vi "Determine Clicked Array Element Index - Determine Array and Scrollbar Properties.vi"(8 "error in (no error)":errorcluster, 10 "Coords of Click":T1, 11 "Array Reference":refnum<vi>) -> (0 "error out":errorcluster, 1 "Scrollbar Properties":T2, 2 "Array Properties":T5, 3 "dup Array Reference":refnum<vi>, 5 "Array Label":string)   [LabVIEW 2021, in "Arrays.lvlib"]
doc: "Determine Clicked Array Element Index - Determine Array and Scrollbar Properties.vi\n\nDescription:\nThis VI determines multiple properties of the array and scrollbars of the array specified by the Array Reference input.\n\nIf no caption has been created for the array of interest, instruct the user how to correct the issue.\n\nInputs:\nArray Reference - Reference to the array to operate on.\n\nCoords of Click - The screen coordinates of the click within the array. These values are used to determine if the click occurred on the selected item.\n\nerror in - Standard error cluster.\n\nOutputs:\ndup Array Reference - Dup reference to the array to operate on.\n\nArray Properties - Cluster containing the array properties of the array specified by the Array Reference input.\n\nScrollbar Properties - Cluster containing the scrollbar properties of the array specified by the Array Reference input.\n\nerror out - standard error cluster.\n\nDeveloped By:\nMark.ridgley\nMark.Ridgley_LabVIEW.Developer@comcast.net"
uses:
  Arrays.lvlib
  <vilib>/Utility/miscctls.llb/LVBoundsTypeDef.ctl
  <vilib>/Utility/miscctls.llb/LVPositionTypeDef.ctl
  <vilib>/Utility/miscctls.llb/LVPoint32TypeDef.ctl
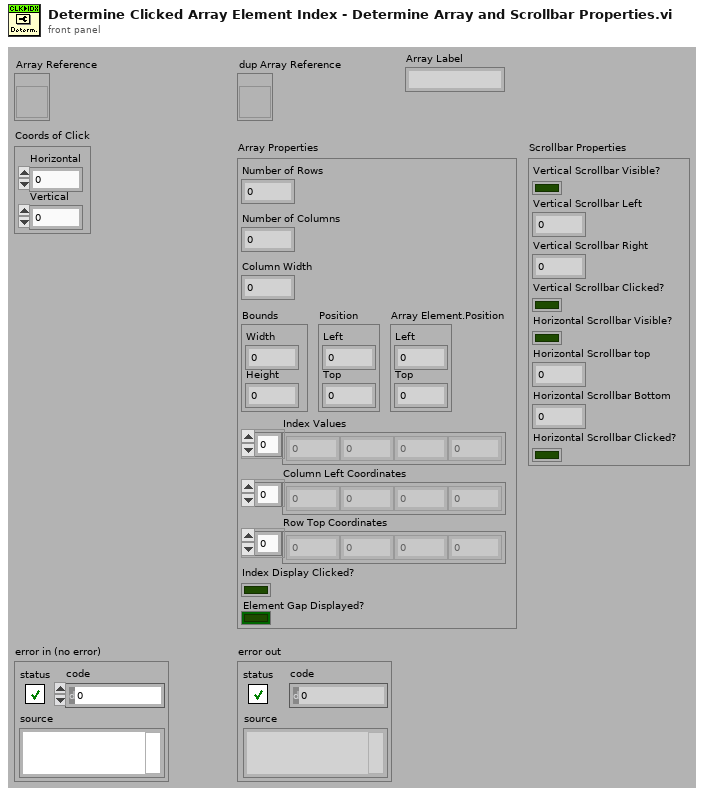
[diagram p1: front panel]
types:
  T1 = typedef "LVPoint32TypeDef.ctl" = cluster{"Horizontal":i32, "Vertical":i32}
  T2 = cluster{"Vertical Scrollbar Visible?":bool, "Vertical Scrollbar Left":i32, "Vertical Scrollbar Right":i32, "Vertical Scrollbar Clicked?":bool, "Horizontal Scrollbar Visible? ":bool, "Horizontal Scrollbar top":i32, "Horizontal Scrollbar Bottom":i32, "Horizontal Scrollbar Clicked?":bool}
  T3 = typedef "LVBoundsTypeDef.ctl" = cluster{"Width":u32, "Height":u32}
  T4 = typedef "LVPositionTypeDef.ctl" = cluster{"Left":i32, "Top":i32}
  T5 = cluster{"Number of Rows":u32, "Number of Columns":u32, "Column Width":u32, "Bounds":T3, "Position":T4, "Array Element.Position":T4, "Index Values":u32[], "Column Left Coordinates":i32[], "Row Top Coordinates":i32[], "Index Display Clicked?":bool, "Element Gap Displayed?":bool}
  T6 = enum16{"Horizontal Scrollbar", "Vertical Scrollbar"}
  T7 = enum16{"Horizontal Scrollbar", "Vertical Scrollbar", "Index Display"}
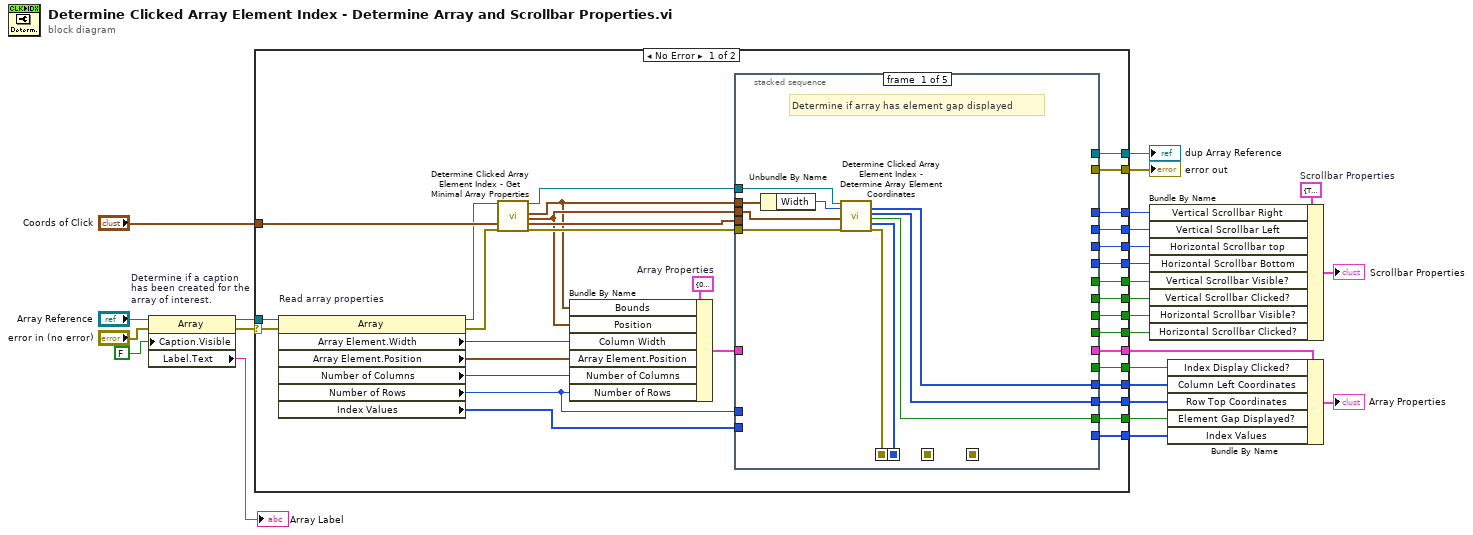
[diagram p0: block diagram]
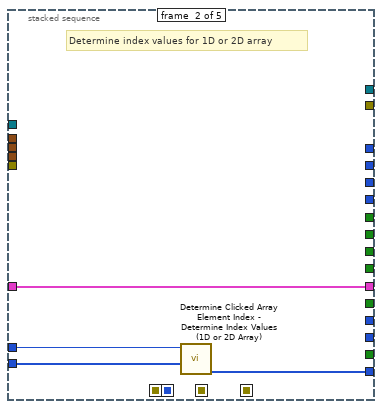
[diagram p2: hidden frame]
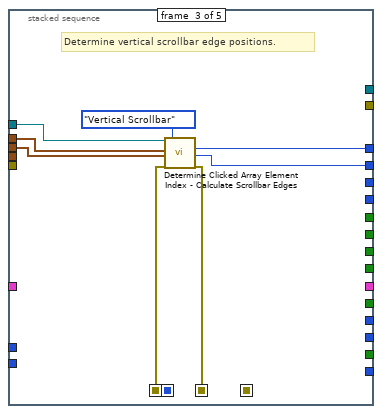
[diagram p3: hidden frame]
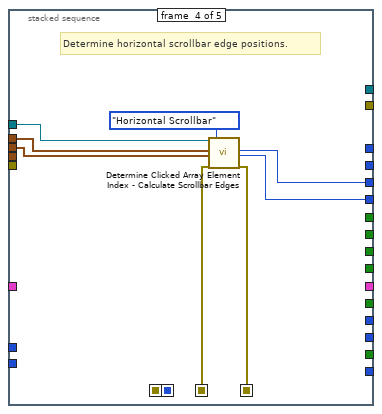
[diagram p4: hidden frame]
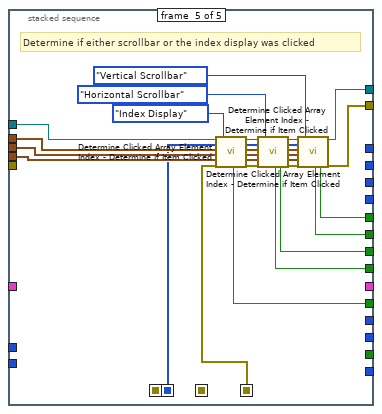
[diagram p5: hidden frame]
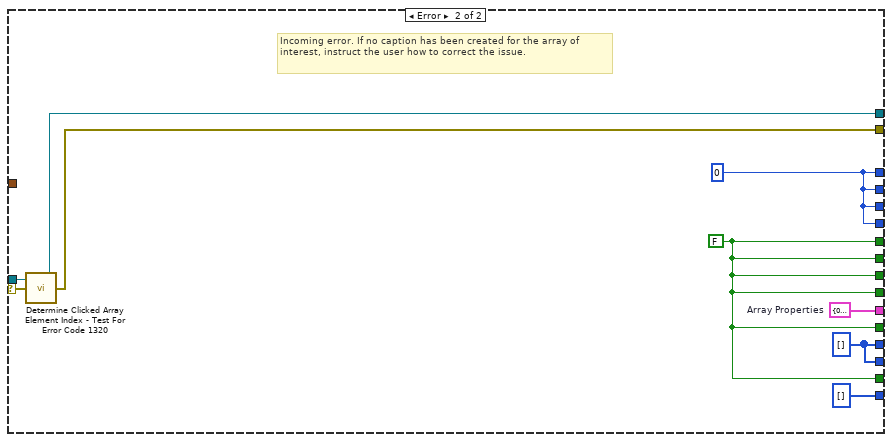
[diagram p6: hidden frame]
diagram:
  w2 = T2 {"Vertical Scrollbar Visible?"=TRUE, "Vertical Scrollbar Left"=0, "Vertical Scrollbar Right"=0, "Vertical Scrollbar Clicked?"=FALSE, "Horizontal Scrollbar Visible? "=TRUE, "Horizontal Scrollbar top"=0, "Horizontal Scrollbar Bottom"=0, "Horizontal Scrollbar Clicked?"=TRUE}  # Scrollbar Properties
  n1 = property on="Determine if a caption has been created for the array of interest." class="Array"(reference="Array Reference", error in="error in (no error)", "Caption.Visible"=FALSE) -> (reference out=w7:refnum<vi>, error out=w8:errorcluster, "Label.Text"=→"Array Label":string)
  n2 = case shown="No Error" w8 {
    selector: w8 -> [w31 w122]
    tunnel: "Coords of Click" -> [w59 _]
    tunnel: [w58 u32[] [] ("Column Left Coordinates")] -> w24
    tunnel: w7 -> [w57 w125]
    tunnel: [w54 w124] -> w23
    tunnel: [w53 w124] -> w22
    tunnel: [w52 w124] -> w21
    tunnel: [w51 w124] -> w20
    tunnel: [w50 w124] -> w19
    tunnel: [w47 w125] -> w18
    tunnel: [w46 w118] -> w17
    tunnel: [w45 w118] -> w16
    tunnel: [w43 w123] -> w15
    tunnel: [w42 w123] -> w14
    tunnel: [w41 w124] -> w13
    tunnel: [w33 w119] -> w12
    tunnel: [w32 w121] -> w11
    tunnel: [w28 w118] -> w4
    tunnel: [w27 w118] -> w3
    frame No Error {
      w29 = T5 {"Number of Rows"=0, "Number of Columns"=0, "Column Width"=0, "Bounds"={"Width"=0, "Height"=0}, "Position"={"Left"=0, "Top"=0}, "Array Element.Position"={"Left"=0, "Top"=0}, "Index Values"=[], "Column Left Coordinates"=[], "Row Top Coordinates"=[], "Index Display Clicked?"=FALSE, "Element Gap Displayed?"=FALSE}  # Array Properties
      n3 = property on="Read array properties" class="Array"(reference=w57, error in=w31) -> (reference out=w55:refnum<vi>, error out=w56:errorcluster, "Array Element.Width"=w30:u32, "Array Element.Position"=w37:T4, "Number of Columns"=w35:u32, "Number of Rows"=w36:u32, "Index Values"=w38:u32[])
      n4 = call "Determine Clicked Array Element Index - Get Minimal Array Properties.vi"("Array Reference"=w55, "Coords of Click"=w59, "error in (no error)"=w56) -> ("dup Array Reference"=w44:refnum<vi>, "Minimal Array Properties.Bounds"=w39:T3, "Minimal Array Properties.Position"=w40:T4, "dup Coords of Click"=w49:T1, "error out"=w48:errorcluster)  [unwired: 12 in]
      n5 = Bundle By Name(cluster=w29, "Bounds"=w39, "Position"=w40, "Column Width"=w30, "Array Element.Position"=w37, "Number of Columns"=w35, "Number of Rows"=w36) -> (w34:T5)
      n6 = stacked-sequence {
        seq-local: [w65 _ _ _ _] -> [_ _ _ _ w93]
        seq-local: [w62 _ _ _ _] -> [_ _ w78 _ _]
        seq-local: [_ _ w77 _ _] -> [_ _ _ w88 _]
        seq-local: [_ _ _ w87 _] -> [_ _ _ _ w90]
        tunnel: [_ w70 _ _ _] -> w58
        tunnel: w38 -> [_ w73 _ _ _]
        tunnel: [_ _ _ _ w114] -> w54
        tunnel: [_ _ _ _ w113] -> w53
        tunnel: [_ _ _ _ w112] -> w52
        tunnel: [_ _ _ _ w111] -> w51
        tunnel: [_ _ _ _ w110] -> w50
        tunnel: w49 -> [_ _ _ _ w97]
        tunnel: w48 -> [w63 _ _ _ _]
        tunnel: [_ _ _ _ w91] -> w47
        tunnel: [_ _ _ _ w92] -> w32
        tunnel: [_ _ w80 _ _] -> w46
        tunnel: [_ _ w79 _ _] -> w45
        tunnel: w39 -> [w61 _ w76 w84 w96]
        tunnel: w36 -> [_ w72 _ _ _]
        tunnel: w40 -> [w64 _ w75 w83 w95]
        tunnel: w44 -> [w69 _ w81 w89 w94]
        tunnel: [w68 _ _ _ _] -> w43
        tunnel: [w67 _ _ _ _] -> w42
        tunnel: [w66 _ _ _ _] -> w41
        tunnel: w34 -> [_ w71 _ _ _]
        tunnel: [_ w71 _ _ _] -> w33
        tunnel: [_ _ _ w86 _] -> w28
        tunnel: [_ _ _ w85 _] -> w27
        frame #0 {
          # "Determine if array has element gap displayed"
          n7 = Unbundle By Name(w61) -> ("Width"=w60:u32)
          n8 = call "Determine Clicked Array Element Index - Determine Array Element Coordinates.vi"("Array Reference"=w69, "Minimal Array Properties.Bounds.Width"=w60, "Minimal Array Properties.Position"=w64, "error in (no error)"=w63) -> ("Column Left Coordinates"=w68:i32[], "Row Top Coordinates"=w67:i32[], "Array has element gap?"=w66:bool, "Un-gapped left coordinates"=w65:i32[], "error out"=w62:errorcluster)  [unwired: 10 in, 1 out]
        }
        frame #1 {
          # "Determine index values for 1D or 2D array"
          n9 = call "Determine Clicked Array Element Index - Determine Index Values (1D or 2D Array).vi"("Array Property.Index Values"=w73, "Array Property.Number of Rows"=w72) -> ("Index Values (1D or 2D Array)"=w70:u32[])  [unwired: 9 in]
        }
        frame #2 {
          # "Determine vertical scrollbar edge positions."
          n10 = call "Determine Clicked Array Element Index - Calculate Scrollbar Edges.vi"("Array Reference"=w81, "Minimal Array Properties.Bounds"=w76, "Minimal Array Properties.Position"=w75, "error in (no error)"=w78, "Select Item"=T6."Vertical Scrollbar") -> ("Minimum Scrollbar Edge"=w79:i32, "Maximum Scrollbar Edge"=w80:i32, "error out"=w77:errorcluster)  [unwired: 11 in, 1 out]
        }
        frame #3 {
          # "Determine horizontal scrollbar edge positions."
          n11 = call "Determine Clicked Array Element Index - Calculate Scrollbar Edges.vi"("Array Reference"=w89, "Minimal Array Properties.Bounds"=w84, "Minimal Array Properties.Position"=w83, "error in (no error)"=w88, "Select Item"=T6."Horizontal Scrollbar") -> ("Minimum Scrollbar Edge"=w86:i32, "Maximum Scrollbar Edge"=w85:i32, "error out"=w87:errorcluster)  [unwired: 11 in, 1 out]
        }
        frame #4 {
          # "Determine if either scrollbar or the index display was clicked"
          n12 = call "Determine Clicked Array Element Index - Determine if Item Clicked.vi"("Array Reference"=w94, "Un-gapped left coordinates"=w93, "Minimal Array Properties.Bounds"=w96, "Minimal Array Properties.Position"=w95, "Coords of Click"=w97, "error in (no error)"=w90, "Select Item"=T7."Index Display") -> ("Item Clicked?"=w114:bool, "dup Array Reference"=w117:refnum<vi>, "dup Un-gapped left coordinates"=w102:i32[], "dup Minimal Array Properties.Bounds"=w108:T3, "dup Minimal Array Properties.Position"=w104:T4, "dup Coords of Click"=w103:T1, "error out"=w109:errorcluster)  [unwired: 5 in, 1 out]
          n13 = call "Determine Clicked Array Element Index - Determine if Item Clicked.vi"("Array Reference"=w117, "Un-gapped left coordinates"=w102, "Minimal Array Properties.Bounds"=w108, "Minimal Array Properties.Position"=w104, "Coords of Click"=w103, "error in (no error)"=w109, "Select Item"=T7."Horizontal Scrollbar") -> ("Item Clicked?"=w113:bool, "Item Visible?"=w112:bool, "dup Array Reference"=w116:refnum<vi>, "dup Un-gapped left coordinates"=w101:i32[], "dup Minimal Array Properties.Bounds"=w107:T3, "dup Minimal Array Properties.Position"=w106:T4, "dup Coords of Click"=w105:T1, "error out"=w115:errorcluster)  [unwired: 5 in]
          n14 = call "Determine Clicked Array Element Index - Determine if Item Clicked.vi"("Array Reference"=w116, "Un-gapped left coordinates"=w101, "Minimal Array Properties.Bounds"=w107, "Minimal Array Properties.Position"=w106, "Coords of Click"=w105, "error in (no error)"=w115, "Select Item"=T7."Vertical Scrollbar") -> ("Item Clicked?"=w111:bool, "Item Visible?"=w110:bool, "dup Array Reference"=w91:refnum<vi>, "error out"=w92:errorcluster)  [unwired: 5 in, 4 out]
        }
      }
    }
    frame Error {
      w119 = T5 {"Number of Rows"=0, "Number of Columns"=0, "Column Width"=0, "Bounds"={"Width"=0, "Height"=0}, "Position"={"Left"=0, "Top"=0}, "Array Element.Position"={"Left"=0, "Top"=0}, "Index Values"=[], "Column Left Coordinates"=[], "Row Top Coordinates"=[], "Index Display Clicked?"=FALSE, "Element Gap Displayed?"=FALSE}  # Array Properties
      w123 = i32[] [] ("Column Left Coordinates")
      w118 = 0 ("Vertical Scrollbar Right")
      w124 = FALSE ("Item Visible?")
      # "Incoming error. If no caption has been created for the array of interest, instruct the user how to correct the issue."
      n15 = call "Determine Clicked Array Element Index - Test For Error Code 1320.vi"("error in"=w122) -> ("error out"=w121:errorcluster)  [unwired: 14 in]
    }
  }
  "error out" <- w11
  "dup Array Reference" <- w18
  n16 = Bundle By Name(cluster=w2, "Vertical Scrollbar Right"=w16, "Vertical Scrollbar Left"=w17, "Horizontal Scrollbar top"=w4, "Horizontal Scrollbar Bottom"=w3, "Vertical Scrollbar Visible?"=w19, "Vertical Scrollbar Clicked?"=w20, "Horizontal Scrollbar Visible?"=w21, "Horizontal Scrollbar Clicked?"=w22) -> (→"Scrollbar Properties":T2)
  n17 = Bundle By Name(cluster=w12, "Index Display Clicked?"=w23, "Column Left Coordinates"=w15, "Row Top Coordinates"=w14, "Element Gap Displayed?"=w13, "Index Values"=w24) -> (→"Array Properties":T5)
